vi "LED_quickPREDICT.vi"() -> ()   [LabVIEW 2012]
uses:
  <vilib>/gmath/NI_Gmath.lvlib
panel:
  out "p_CE(cd/A_":dbl format="%_5e"
  out "p_Lum":dbl format="%_5e"
  out "p_Jden(mA/cm2)":dbl format="%_5e"
  out "p_I(A)":dbl format="%_5e"
  out "p_V(V)":dbl format="%_5e"
  out "Index":i32
  in  "target Lum(cd/m2)":dbl=100.0
  out "current density array":dbl[](array[numeric])
  out "CE array":dbl[](array[numeric])
  out "Candela array":dbl[](array[numeric]) format="%_6g"
  out "Luminance array":dbl[](array[numeric]) format="%_6g"
  out "Current array":dbl[](array[numeric]) format="%_6g"
  in  "Method":i32(ring)=3 items=["nearest", "linear", "spline", "cubic Hermite", "Lagrange"]
  out "V Array":dbl[](array[numeric])
  out "Vi":dbl
  out "step":dbl
  in  "Interpolation size":i32=1001
  out "Current Efficiency vs Luminance/Current Density":cluster{"Y":dbl[], "Y":dbl[]}[](graph)
  out "Current Density/Luminance vs Voltage":cluster{"Y":dbl[], "Y":dbl[]}[](graph)
  out "current efficiency (Cd/A)":dbl[](array[numeric])
  out "current density (mA/cm2)":dbl[](array[numeric])
  in  "DeviceArea(m2)":dbl=3e-06
  out "uW":dbl[](array[numeric])
  out "luminance (Cd/m2)":dbl[](array[numeric])
  out "candela (Cd)":dbl[](array[numeric])
  out "array":dbl[][](array[numeric])
  out "substring":string
  out "current":dbl[](array[numeric])=[6.47737e-06, 2.6904e-06, 1.39949e-05, 2.68063e-06, 9.1124e-06, 1.90109e-14, 1.97383e-05, 3.27886e-05, 1.52434e-14, 1.39406e-14, 1.38211e-06, 5.60771e-06, 1.05119e-14, 5.17343e-06, 8.75954e-15, 7.94526e-06, 3.52097e-06, 6.93229e-15, 6.13103e-06, 2.17143e-06, 5.79229e-15, 4.74349e-06, 1.31046e-05, 1.46246e-05, 1.64051e-05, 7.16029e-06, 1.45269e-05, 1.8848e-05, 1.69046e-05, 2.94011e-05, 3.6784e-05, 4.04863e-05, 4.8336e-05, 7.44474e-05, 8.9224e-05, 0.00011096, 0.000158297, 0.000223114, 0.000309646, 0.000425274, 0.00055936, 0.00072124, 0.000872154, 0.00098648, 0.00107, 0.00113, 0.00114, 0.00113, 0.00111, 0.00107, 0.00102, 0.000982897, 0.000954886, 0.00092416, 0.000901903, 0.000883446, 0.000877257, 0.000876606, 0.000867594, 0.00086716, 0.00086032, 0.000838063, 0.000814503, 0.000782583, 0.000746537, 0.000713966, 0.000685194, 0.000641549, 0.00060116, 0.000566634, 0.00053808, 0.00051224, 0.000480646, 0.000459474, 0.000436566, 0.000413983, 0.000402691, 0.000382714, 0.0003648, 0.000347754, 0.000340697, 0.000318657, 0.000305303, 0.000288366, 0.000271103, 0.000258183, 0.000245046, 0.000230497, 0.00021584, 0.000209109, 0.000197383, 0.000185223, 0.000174909, 0.000168069, 0.000157211, 0.000145051, 0.00014288, 0.000137777, 0.000130069, 0.000120731, 0.000116931, 0.00011324, 0.000107421, 9.73017e-05, 9.4924e-05, 8.8844e-05, 8.98971e-05, 8.97126e-05, 7.89206e-05, 7.94309e-05, 7.32097e-05, 6.66629e-05, 6.16903e-05, 5.57949e-05, 6.20811e-05, 5.63594e-05, 5.13543e-05, 4.87377e-05, 4.47097e-05, 4.64794e-05, 4.35371e-05, 4.20389e-05, 4.2408e-05, 3.41891e-05, 3.3744e-05, 3.43086e-05, 3.08126e-05, 3.16377e-05, 3.192e-05, 3.3744e-05, 2.9792e-05, 2.53949e-05, 2.44829e-05, 2.15949e-05, 1.91954e-05, 2.39617e-05, 2.4244e-05, 2.0216e-05, 1.47983e-05, 1.92823e-05, 1.94777e-05, 1.04098e-05, 1.98794e-05, 1.80771e-05, 1.34303e-05, 1.30177e-05, 1.81314e-05, 1.28549e-05, 1.38971e-05, 1.89891e-05, 1.748e-05, 1.85766e-05, 1.28983e-05, 8.3524e-06, 7.15051e-06, 6.38943e-06, 1.80337e-05, 1.7784e-05, 8.00931e-06, 1.04055e-05, 1.15629e-05, 3.42869e-06, 7.79109e-06, 1.20514e-05, 6.23526e-06, 5.57297e-06, 1.03979e-05, 9.60097e-06, 3.77611e-06, 4.99971e-06, 1.86091e-05, 7.97783e-06, 4.75326e-06, 1.34954e-05, 4.08663e-06, 5.80206e-06, 8.21669e-06, 3.33531e-06, 5.61531e-06, 6.92903e-06, 6.47954e-06, 5.80206e-06, 3.11817e-06, 7.95177e-06, 1.47983e-05, 1.30177e-05, 4.10617e-06, 1.09766e-06, 1.23337e-14, 4.39606e-06, 2.204e-06, 3.85646e-06, 1.12371e-05, 2.84674e-06, 1.52e-14, 1.57537e-14, 1.62097e-14, 1.67526e-05, 1.65789e-14, 3.78263e-06, 6.14189e-06]
  out "voltage":dbl[](array[numeric])=[380.0, 382.0, 384.0, 386.0, 388.0, 390.0, 392.0, 394.0, 396.0, 398.0, 400.0, 402.0, 404.0, 406.0, 408.0, 410.0, 412.0, 414.0, 416.0, 418.0, 420.0, 422.0, 424.0, 426.0, 428.0, 430.0, 432.0, 434.0, 436.0, 438.0, 440.0, 442.0, 444.0, 446.0, 448.0, 450.0, 452.0, 454.0, 456.0, 458.0, 460.0, 462.0, 464.0, 466.0, 468.0, 470.0, 472.0, 474.0, 476.0, 478.0, 480.0, 482.0, 484.0, 486.0, 488.0, 490.0, 492.0, 494.0, 496.0, 498.0, 500.0, 502.0, 504.0, 506.0, 508.0, 510.0, 512.0, 514.0, 516.0, 518.0, 520.0, 522.0, 524.0, 526.0, 528.0, 530.0, 532.0, 534.0, 536.0, 538.0, 540.0, 542.0, 544.0, 546.0, 548.0, 550.0, 552.0, 554.0, 556.0, 558.0, 560.0, 562.0, 564.0, 566.0, 568.0, 570.0, 572.0, 574.0, 576.0, 578.0, 580.0, 582.0, 584.0, 586.0, 588.0, 590.0, 592.0, 594.0, 596.0, 598.0, 600.0, 602.0, 604.0, 606.0, 608.0, 610.0, 612.0, 614.0, 616.0, 618.0, 620.0, 622.0, 624.0, 626.0, 628.0, 630.0, 632.0, 634.0, 636.0, 638.0, 640.0, 642.0, 644.0, 646.0, 648.0, 650.0, 652.0, 654.0, 656.0, 658.0, 660.0, 662.0, 664.0, 666.0, 668.0, 670.0, 672.0, 674.0, 676.0, 678.0, 680.0, 682.0, 684.0, 686.0, 688.0, 690.0, 692.0, 694.0, 696.0, 698.0, 700.0, 702.0, 704.0, 706.0, 708.0, 710.0, 712.0, 714.0, 716.0, 718.0, 720.0, 722.0, 724.0, 726.0, 728.0, 730.0, 732.0, 734.0, 736.0, 738.0, 740.0, 742.0, 744.0, 746.0, 748.0, 750.0, 752.0, 754.0, 756.0, 758.0, 760.0, 762.0, 764.0, 766.0, 768.0, 770.0, 772.0, 774.0, 776.0, 778.0, 780.0]
  in  "file (use dialog)":path
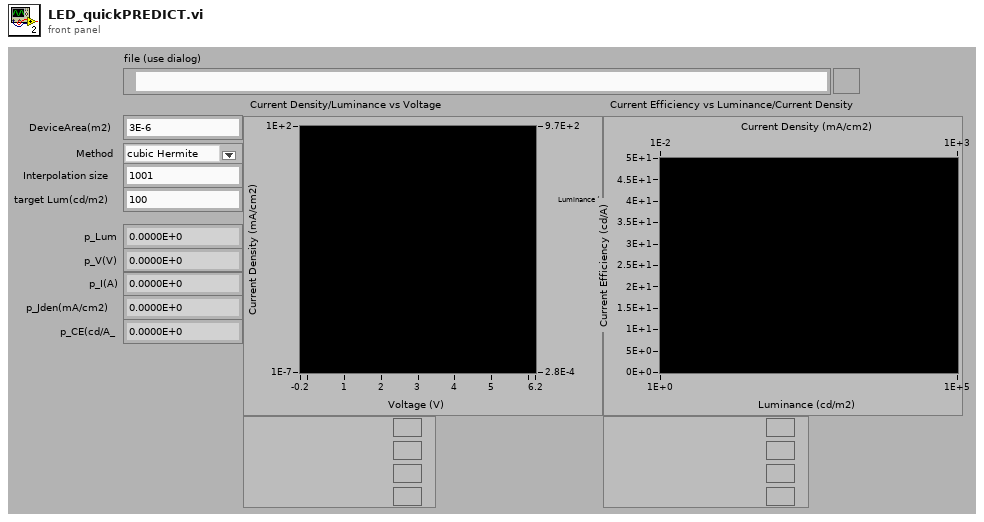
[diagram p1: front panel]
types:
  T1 = cluster{"luminance (Cd/m2)":dbl[], "current efficiency (Cd/A)":dbl[]}
  T2 = cluster{"current density (mA/cm2)":dbl[], "current efficiency (Cd/A)":dbl[]}
  T3 = cluster{"Luminance array":dbl[], "CE array":dbl[]}
  T4 = cluster{"current density array":dbl[], "CE array":dbl[]}
  T5 = cluster{"current density array":dbl[], "CE array":dbl[]}[]
  T6 = cluster{"voltage":dbl[], "luminance (Cd/m2)":dbl[]}
  T7 = cluster{"V Array":dbl[], "Luminance array":dbl[]}
  T8 = cluster{"V Array":dbl[], "Luminance array":dbl[]}[]
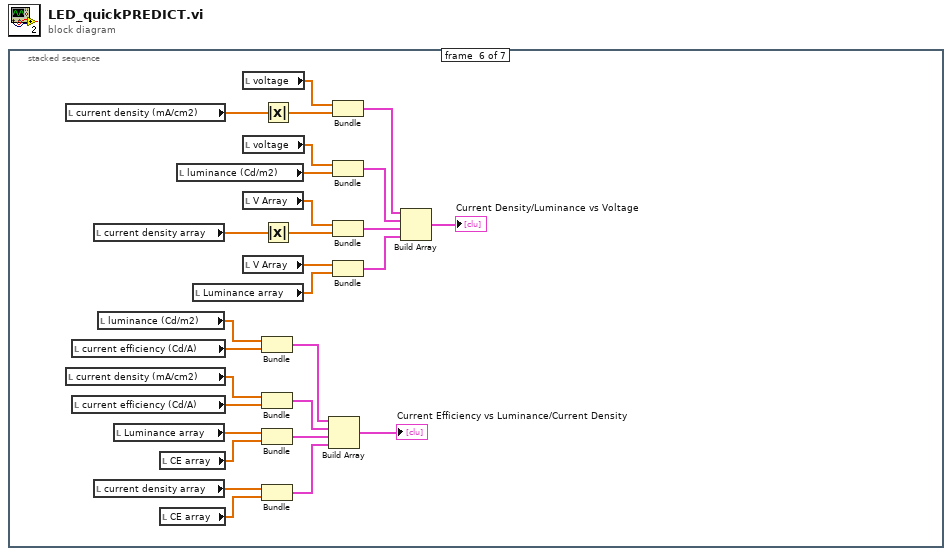
[diagram p0: block diagram]
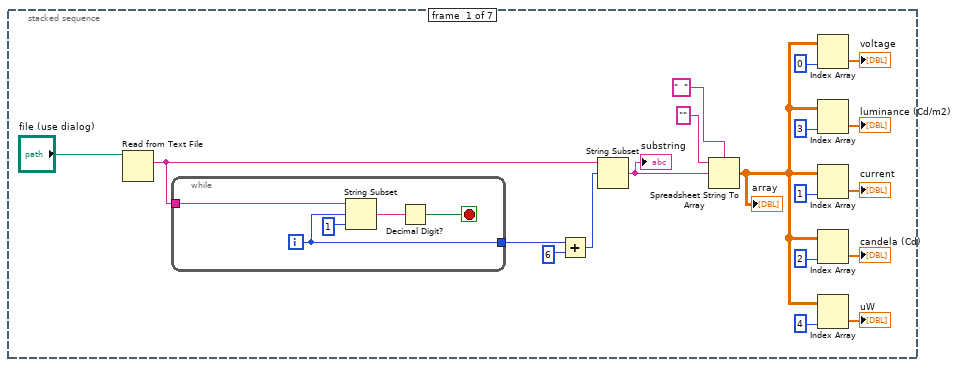
[diagram p2: hidden frame]
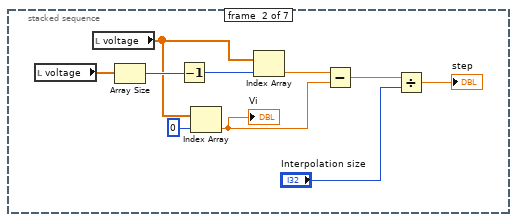
[diagram p3: hidden frame]
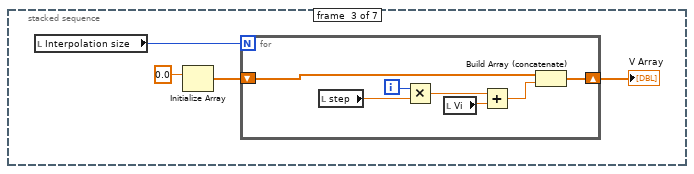
[diagram p4: hidden frame]
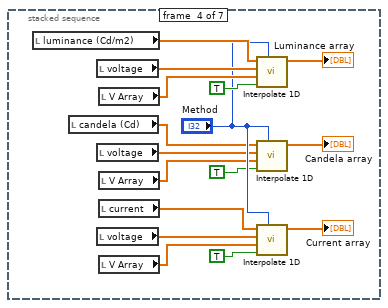
[diagram p5: hidden frame]
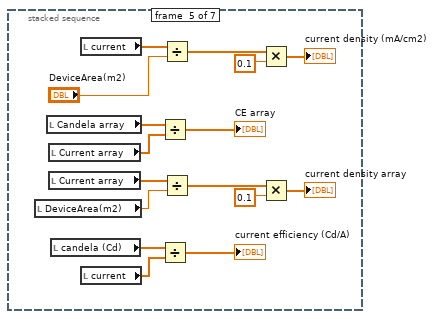
[diagram p6: hidden frame]
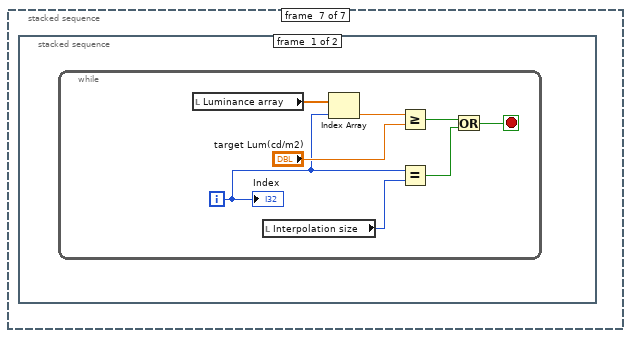
[diagram p7: hidden frame]
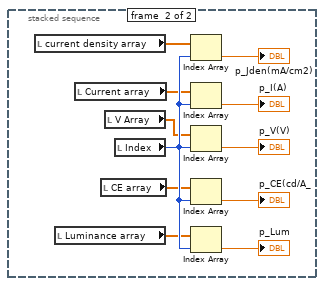
[diagram p8: hidden frame]
diagram:
  n1 = stacked-sequence {
    frame #0 {
      n2 = Read from Text File(file (use dialog)="file (use dialog)") -> (text=w15:string)  [unwired: 3 in, 3 out]
      n3 = while {
        tunnel: w15 -> [w24]
        tunnel: [w20] -> w12
        i -> [w20]
        stop <- w21 stop-if-true
        n4 = String Subset(string=w24, offset (0)=w20, length (rest)=1 ("length (rest)")) -> (substring=w22:string)
        n5 = Decimal Digit?(1:w22) -> (0:w21:bool)
      }
      n6 = Add(x=w12, y=6) -> (x+y=w10:i32)
      n7 = String Subset(string=w15, offset (0)=w10) -> (substring=w13:string)  [unwired: 1 in]
      "substring" <- w13
      n8 = Spreadsheet String To Array(delimiter (Tab)="  ", format string="", spreadsheet string=w13) -> (array=w1:dbl[][])  [unwired: 1 in]
      "array" <- w1
      n9 = Index Array(array=w1, index (col)=0 ("disabled index (col)")) -> (element=→"voltage":dbl[])  [unwired: 1 in]
      n10 = Index Array(array=w1, index (col)=3 ("disabled index (col)")) -> (element=→"luminance (Cd/m2)":dbl[])  [unwired: 1 in]
      n11 = Index Array(array=w1, index (col)=1 ("disabled index (col)")) -> (element=→"current":dbl[])  [unwired: 1 in]
      n12 = Index Array(array=w1, index (col)=2 ("disabled index (col)")) -> (element=→"candela (Cd)":dbl[])  [unwired: 1 in]
      n13 = Index Array(array=w1, index (col)=4 ("disabled index (col)")) -> (element=→"uW":dbl[])  [unwired: 1 in]
    }
    frame #1 {
      n14 = local read "voltage"() -> (w34:dbl[])
      n15 = local read "voltage"() -> (w30:dbl[])
      n16 = Array Size(array=w34) -> (size(s)=w33:i32)
      n17 = Decrement(x=w33) -> (x-1=w31:i32)
      n18 = Index Array(array=w30, index=0) -> (element=w25:dbl)
      "Vi" <- w25
      n19 = Index Array(array=w30, index=w31) -> (element=w29:dbl)
      n20 = Subtract(x=w29, y=w25) -> (x-y=w28:dbl)
      n21 = Divide(x=w28, y="Interpolation size") -> (x/y=→"step":dbl)
    }
    frame #2 {
      n22 = local read "Interpolation size"() -> (w38:i32)
      n23 = Initialize Array(0.0 ("element")) -> (w36:dbl[])  [unwired: 1 in]
      n24 = for {
        N: w38 -> [_]
        shift-right: [w39] -> w35
        shift-left: w36 -> [w40]
        i -> [w42]
        n25 = local read "step"() -> (w43:dbl)
        n26 = Multiply(x=w42, y=w43) -> (x*y=w45:dbl)
        n27 = local read "Vi"() -> (w44:dbl)
        n28 = Add(x=w45, y=w44) -> (x+y=w41:dbl)
        n29 = Build Array (concatenate)(w40, w41) -> (w39:dbl[])
      }
      "V Array" <- w35
    }
    frame #3 {
      n30 = local read "luminance (Cd/m2)"() -> (w54:dbl[])
      n31 = local read "candela (Cd)"() -> (w50:dbl[])
      n32 = local read "voltage"() -> (w55:dbl[])
      n33 = local read "voltage"() -> (w49:dbl[])
      n34 = local read "voltage"() -> (w60:dbl[])
      n35 = local read "V Array"() -> (w56:dbl[])
      n36 = local read "V Array"() -> (w48:dbl[])
      n37 = local read "current"() -> (w59:dbl[])
      n38 = local read "V Array"() -> (w61:dbl[])
      n39 = call <vilib>:"Interpolate 1D.vi"("method"="Method", "X is monotonic"=TRUE, "xi"=w56, "X"=w55, "Y"=w54) -> ("yi"=→"Luminance array":dbl[])  [unwired: 4 in, 2 out]
      n40 = call <vilib>:"Interpolate 1D.vi"("method"="Method", "X is monotonic"=TRUE, "xi"=w48, "X"=w49, "Y"=w50) -> ("yi"=→"Candela array":dbl[])  [unwired: 4 in, 2 out]
      n41 = call <vilib>:"Interpolate 1D.vi"("method"="Method", "X is monotonic"=TRUE, "xi"=w61, "X"=w60, "Y"=w59) -> ("yi"=→"Current array":dbl[])  [unwired: 4 in, 2 out]
    }
    frame #4 {
      n42 = local read "DeviceArea(m2)"() -> (w67:dbl)
      n43 = local read "Candela array"() -> (w65:dbl[])
      n44 = local read "Current array"() -> (w66:dbl[])
      n45 = local read "Current array"() -> (w63:dbl[])
      n46 = local read "candela (Cd)"() -> (w72:dbl[])
      n47 = local read "current"() -> (w70:dbl[])
      n48 = local read "current"() -> (w73:dbl[])
      n49 = Divide(x=w65, y=w66) -> (x/y=→"CE array":dbl[])
      n50 = Divide(x=w72, y=w73) -> (x/y=→"current efficiency (Cd/A)":dbl[])
      n51 = Divide(x=w70, y="DeviceArea(m2)") -> (x/y=w75:dbl[])
      n52 = Divide(x=w63, y=w67) -> (x/y=w68:dbl[])
      n53 = Multiply(x=w75, y=0.1) -> (x*y=→"current density (mA/cm2)":dbl[])
      n54 = Multiply(x=w68, y=0.1) -> (x*y=→"current density array":dbl[])
    }
    frame #5 {
      n55 = local read "current density (mA/cm2)"() -> (w99:dbl[])
      n56 = local read "current density (mA/cm2)"() -> (w93:dbl[])
      n57 = local read "current efficiency (Cd/A)"() -> (w91:dbl[])
      n58 = local read "current efficiency (Cd/A)"() -> (w92:dbl[])
      n59 = local read "current density array"() -> (w79:dbl[])
      n60 = local read "current density array"() -> (w88:dbl[])
      n61 = local read "luminance (Cd/m2)"() -> (w100:dbl[])
      n62 = local read "Luminance array"() -> (w89:dbl[])
      n63 = local read "CE array"() -> (w90:dbl[])
      n64 = local read "CE array"() -> (w87:dbl[])
      n65 = local read "luminance (Cd/m2)"() -> (w103:dbl[])
      n66 = local read "Luminance array"() -> (w84:dbl[])
      n67 = local read "voltage"() -> (w94:dbl[])
      n68 = local read "voltage"() -> (w104:dbl[])
      n69 = local read "V Array"() -> (w82:dbl[])
      n70 = local read "V Array"() -> (w83:dbl[])
      n71 = Bundle("luminance (Cd/m2)"=w100, "current efficiency (Cd/A)"=w91) -> (w95:T1)  [unwired: 1 in]
      n72 = Bundle("current density (mA/cm2)"=w93, "current efficiency (Cd/A)"=w92) -> (w96:T2)  [unwired: 1 in]
      n73 = Bundle("Luminance array"=w89, "CE array"=w90) -> (w86:T3)  [unwired: 1 in]
      n74 = Bundle("current density array"=w88, "CE array"=w87) -> (w85:T4)  [unwired: 1 in]
      n75 = Absolute Value(x=w99) -> (abs(x)=w105:dbl[])
      n76 = Absolute Value(x=w79) -> (abs(x)=w78:dbl[])
      n77 = Build Array(w95, w96, w86, w85) -> (→"Current Efficiency vs Luminance/Current Density":T5)
      n78 = Bundle("voltage"=w94, w105) -> (w101:cluster{"voltage":dbl[], dbl[]})  [unwired: 1 in]
      n79 = Bundle("voltage"=w104, "luminance (Cd/m2)"=w103) -> (w102:T6)  [unwired: 1 in]
      n80 = Bundle("V Array"=w82, w78) -> (w81:cluster{"V Array":dbl[], dbl[]})  [unwired: 1 in]
      n81 = Bundle("V Array"=w83, "Luminance array"=w84) -> (w80:T7)  [unwired: 1 in]
      n82 = Build Array(w101, w102, w81, w80) -> (→"Current Density/Luminance vs Voltage":T8)
    }
    frame #6 {
      n83 = stacked-sequence {
        frame #0 {
          n84 = while {
            i -> [w108]
            stop <- w106 stop-if-true
            n85 = local read "Luminance array"() -> (w112:dbl[])
            n86 = local read "Interpolation size"() -> (w107:i32)
            n87 = Index Array(array=w112, index=w108) -> (element=w111:dbl)
            n88 = Greater Or Equal?(x=w111, y="target Lum(cd/m2)") -> (x >= y?=w110:bool)
            n89 = Equal?(x=w108, y=w107) -> (x = y?=w109:bool)
            n90 = Or(x=w110, y=w109) -> (x .or. y?=w106:bool)
            "Index" <- w108
          }
        }
        frame #1 {
          n91 = local read "current density array"() -> (w121:dbl[])
          n92 = local read "Luminance array"() -> (w122:dbl[])
          n93 = local read "Current array"() -> (w120:dbl[])
          n94 = local read "CE array"() -> (w123:dbl[])
          n95 = local read "V Array"() -> (w119:dbl[])
          n96 = local read "Index"() -> (w124:i32)
          n97 = Index Array(array=w121, index=w124) -> (element=→"p_Jden(mA/cm2)":dbl)
          n98 = Index Array(array=w120, index=w124) -> (element=→"p_I(A)":dbl)
          n99 = Index Array(array=w119, index=w124) -> (element=→"p_V(V)":dbl)
          n100 = Index Array(array=w123, index=w124) -> (element=→"p_CE(cd/A_":dbl)
          n101 = Index Array(array=w122, index=w124) -> (element=→"p_Lum":dbl)
        }
      }
    }
  }
